vi "IP9258_POWER_ON_WebSwitch.vi"() -> ()   [LabVIEW 2011]
doc: "Example of using standard HTTP protocol for recieving a web site (the HTML source)\n\n\nThis example uses the GET command. For general information about the HTTP protocol and other commands go to\nhttp://www.w3.org/Protocols\n\n\nBjornar Svingen\nbjornar.svingen@sintef.no bjornar.svingen@ktv.no"
uses:
  <vilib>/addons/internet/telnet/telnet.llb/Telnet Session.ctl
  <vilib>/addons/internet/NI_InternetTK_Core_VIs.lvlib
panel:
  out "PowerOn CMD":string
  out "log3":string
  out "log2":string
  out "telnet connection":T1
  out "log1":string
  out "DebugView":string
  out "Begin Time":u32
  # "IP9258 Power On"
  # "2014-8-26"
  # "本程式是Telnet方式來控制IP9258\n1.Windows 需開啟Telnet 服務( Need eable Telnet Client Service)\n2.IP_POWER_WEB_SWITCH_IP=?;       /* need define it /\n3.IP9258_ACCOUNT_PASSWORD=?; /* need define it */\n4.IP9258_POWER-ON_CMD=1111; /* 可自行定義 要ON或Off ,1=0n ,0=off */"
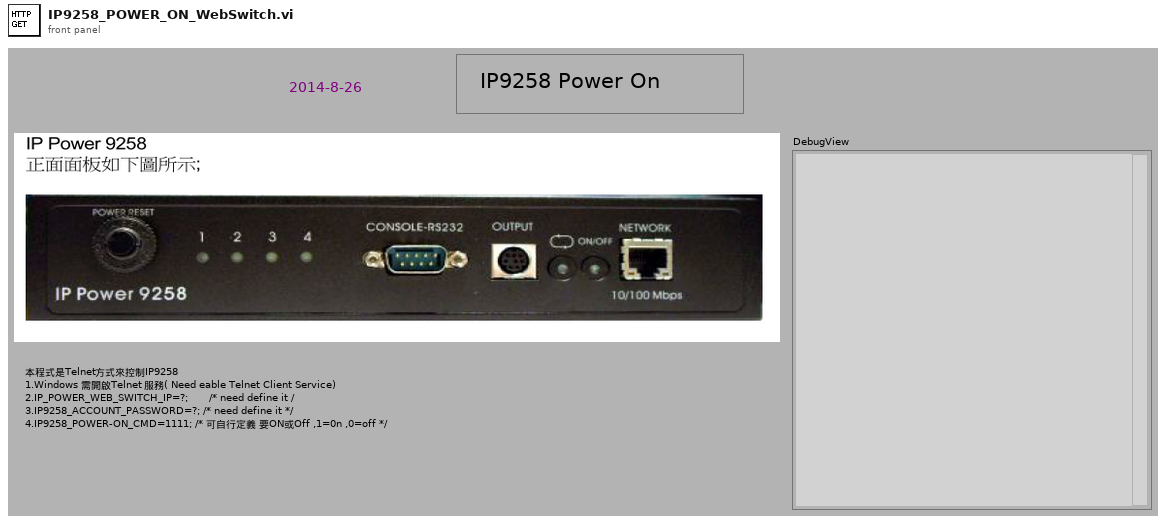
[diagram p1: front panel]
types:
  T1 = typedef "Telnet Session.ctl" = refnum<k1>
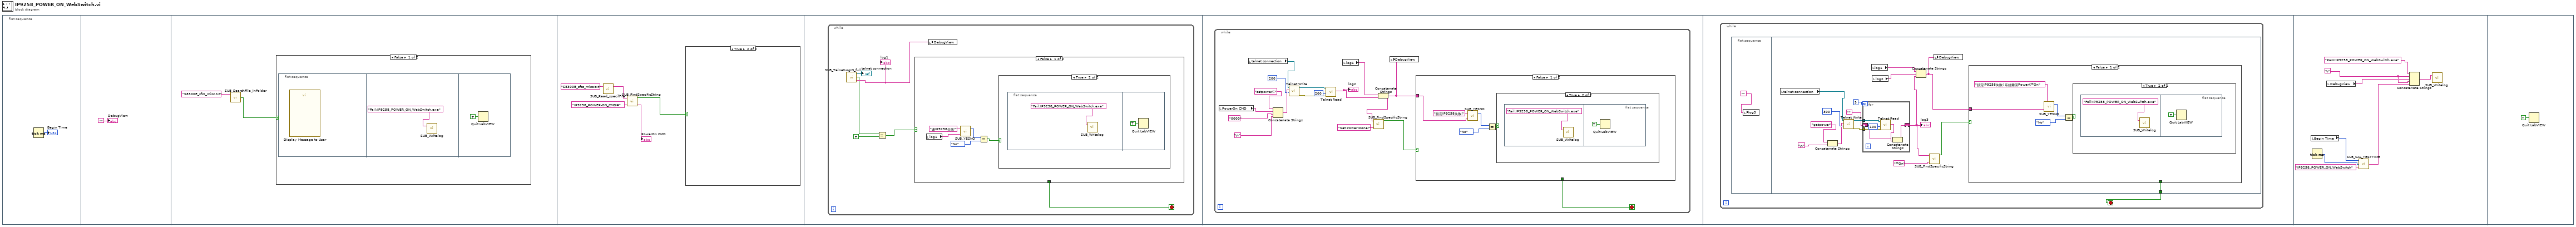
[diagram p0: block diagram]
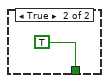
[diagram p5: hidden frame]
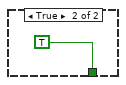
[diagram p7: hidden frame]
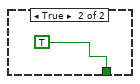
[diagram p9: hidden frame]
diagram:
  n1 = flat-sequence {
    frame #0 {
      n2 = Tick Count (ms)() -> (millisecond timer value=→"Begin Time":u32)
    }
    frame #1 {
      "DebugView" <- ""
    }
    frame #2 {
      n3 = call "SUB_SearchFile_inFolder.vi"("Search Filename in Folder"="S8300E_sfcs_misc.txt" ("name or relative path")) -> ("File Existing True/Flase"=w3:bool)  [unwired: 1 in]
      n4 = case shown="False" w3 {
        frame False {
          n5 = flat-sequence {
            frame #0 {
              n6 = call "Display Message to User"() -> ()  [unwired: 10 in, 2 out]
            }
            frame #1 {
              n7 = call "SUB_Writelog.vi"("Pass/Fail"="Fail:IP9258_POWER_ON_WebSwitch.exe") -> ()  [unwired: 2 in]
            }
            frame #2 {
              n8 = Quit LabVIEW(quit? (T)=TRUE) -> ()
            }
          }
        }
        frame True {
        }
      }
    }
    frame #3 {
      n9 = call "SUB_Read_specifFile.vi"("name or relative path"="S8300E_sfcs_misc.txt") -> ("text"=w10:string)  [unwired: 1 in, 1 out]
      n10 = call "SUB_FindSpecificString.vi"("Find this String"="IP9258_POWER-ON_CMD=", "String data"=w10) -> ("before \"; \" string"=→"PowerOn CMD":string, "Found"=w8:bool)  [unwired: 2 in]
      n11 = case shown="True" w8 {
        frame False {
        }
        frame True {
        }
      }
    }
    frame #4 {
      n12 = while {
        stop <- w13 stop-if-true
        n13 = call "SUB_TelnetLogIN_full.vi"() -> ("telnet connection"=→"telnet connection":T1, "Pass ?"=w16:bool, "data out"=w17:string)  [unwired: 2 in]
        "log1" <- w17
        n14 = Equal?(x=w16, y=TRUE) -> (x = y?=w14:bool)
        n15 = case shown="False" w14 {
          tunnel: [_ TRUE] -> w13
          frame False {
            n16 = local read "log1"() -> (w22:string)
            n17 = call "SUB_YESNO.vi"("Debug View"=w22, "Status"="連IP9258失敗!") -> ("yes/no"=w20:enum32{"No Selection", "Yes", "No", "None"})  [unwired: 1 in]
            n18 = Equal?(x=w20, y=enum32{"No Selection", "Yes", "No", "None"}."No") -> (x = y?=w18:bool)
            n19 = case shown="True" w18 {
              frame False {
              }
              frame True {
                n20 = flat-sequence {
                  frame #0 {
                    n21 = call "SUB_Writelog.vi"("Pass/Fail"="Fail:IP9258_POWER_ON_WebSwitch.exe") -> ()  [unwired: 2 in]
                  }
                  frame #1 {
                    n22 = Quit LabVIEW(quit? (T)=TRUE) -> ()
                  }
                }
              }
            }
          }
          frame True {
          }
        }
        n23 = local write "DebugView"(w17) -> ()
      }
    }
    frame #5 {
      n24 = while {
        stop <- w30 stop-if-true
        n25 = local read "PowerOn CMD"() -> (w28:string)
        n26 = local read "telnet connection"() -> (w41:T1)
        n27 = Concatenate Strings("setpower=" ("data in"), w28, "0000" ("data in"), "\n") -> (w35:string)
        n28 = call <vilib>:"Telnet Write.vi"("timeout ms (25000)"=200, "data in"=w35, "telnet connection"=w41) -> ("error out"=w39:errorcluster, "telnet connection out"=w40:T1)  [unwired: 4 in, 1 out]
        n29 = call <vilib>:"Telnet Read.vi"("error in (no error)"=w39, "timeout ms (25000)"=200, "telnet connection"=w40) -> ("data out"=w37:string)  [unwired: 4 in, 2 out]
        "log2" <- w37
        n30 = local read "log1"() -> (w38:string)
        n31 = Concatenate Strings(w38, w37) -> (w29:string)
        n32 = call "SUB_FindSpecificString.vi"("Find this String"="Set Power Done!", "String data"=w29) -> ("Found"=w31:bool)  [unwired: 2 in, 1 out]
        n33 = local write "DebugView"(w29) -> ()
        n34 = case shown="False" w31 {
          tunnel: [_ TRUE] -> w30
          tunnel: w29 -> [w45 _]
          frame False {
            n35 = call "SUB_YESNO.vi"("Debug View"=w45, "Status"="設定IP9258失敗!") -> ("yes/no"=w43:enum32{"No Selection", "Yes", "No", "None"})  [unwired: 1 in]
            n36 = Equal?(x=w43, y=enum32{"No Selection", "Yes", "No", "None"}."No") -> (x = y?=w42:bool)
            n37 = case shown="True" w42 {
              frame False {
              }
              frame True {
                n38 = flat-sequence {
                  frame #0 {
                    n39 = call "SUB_Writelog.vi"("Pass/Fail"="Fail:IP9258_POWER_ON_WebSwitch.exe") -> ()  [unwired: 2 in]
                  }
                  frame #1 {
                    n40 = Quit LabVIEW(quit? (T)=TRUE) -> ()
                  }
                }
              }
            }
          }
          frame True {
          }
        }
      }
    }
    frame #6 {
      n41 = while {
        stop <- w50 stop-if-true
        n42 = flat-sequence {
          tunnel: [w58] -> w50
          frame #0 {
            n43 = local write "log3"("") -> ()
          }
          frame #1 {
            n44 = local read "telnet connection"() -> (w62:T1)
            n45 = Concatenate Strings("getpower" ("data in"), "\n") -> (w66:string)
            n46 = call <vilib>:"Telnet Write.vi"("timeout ms (25000)"=300, "data in"=w66, "telnet connection"=w62) -> ("error out"=w64:errorcluster, "telnet connection out"=w63:T1)  [unwired: 4 in, 1 out]
            n47 = for {
              N: 5 -> [_]
              tunnel: w64 -> [w72]
              tunnel: w63 -> [w71]
              shift-right: [w69] -> w52
              shift-left: "" -> [w68]
              n48 = call <vilib>:"Telnet Read.vi"("error in (no error)"=w72, "timeout ms (25000)"=100, "telnet connection"=w71) -> ("data out"=w70:string)  [unwired: 4 in, 2 out]
              n49 = Concatenate Strings(w68, w70) -> (w69:string)
            }
            "log3" <- w52
            n50 = local read "log1"() -> (w57:string)
            n51 = local read "log2"() -> (w56:string)
            n52 = Concatenate Strings(w57, w56, w52) -> (w55:string)
            n53 = call "SUB_FindSpecificString.vi"("Find this String"="=On", "String data"=w52) -> ("Found"=w59:bool)  [unwired: 2 in, 1 out]
            n54 = local write "DebugView"(w55) -> ()
            n55 = case shown="False" w59 {
              tunnel: [_ TRUE] -> w58
              tunnel: w55 -> [w74 _]
              frame False {
                n56 = call "SUB_YESNO.vi"("Debug View"=w74, "Status"="設定IP9258失敗! 系統需回PowerX=On") -> ("yes/no"=w76:enum32{"No Selection", "Yes", "No", "None"})  [unwired: 1 in]
                n57 = Equal?(x=w76, y=enum32{"No Selection", "Yes", "No", "None"}."No") -> (x = y?=w75:bool)
                n58 = case shown="True" w75 {
                  frame False {
                  }
                  frame True {
                    n59 = flat-sequence {
                      frame #0 {
                        n60 = call "SUB_Writelog.vi"("Pass/Fail"="Fail:IP9258_POWER_ON_WebSwitch.exe") -> ()  [unwired: 2 in]
                      }
                      frame #1 {
                        n61 = Quit LabVIEW(quit? (T)=TRUE) -> ()
                      }
                    }
                  }
                }
              }
              frame True {
              }
            }
          }
        }
      }
    }
    frame #7 {
      w83 = "\r"
      n62 = local read "Begin Time"() -> (w89:u32)
      n63 = Tick Count (ms)() -> (millisecond timer value=w88:u32)
      n64 = local read "DebugView"() -> (w84:string)
      n65 = call "SUB_CAL_TESTTIME.vi"("Test Item name"="IP9258_POWER_ON_WebSwitch", "Stop tick time"=w88, "Start tick time"=w89) -> ("Test Time output"=w82:string)  [unwired: 2 in]
      n66 = Concatenate Strings("Pass:IP9258_POWER_ON_WebSwitch.exe", w83, w84, w83, w82) -> (w85:string)
      n67 = call "SUB_Writelog.vi"("Pass/Fail"=w85) -> ()  [unwired: 2 in]
    }
    frame #8 {
      n68 = Quit LabVIEW(quit? (T)=TRUE) -> ()
    }
  }
